vi "Scan area calc.vi"(0 "Y Width":dbl, 1 "Major Axis Direction":u16(ring) items=["Positive", "Negative"], 2 "X Width":dbl, 3 "Minor Axis Direction":u16(ring) items=["Positive", "Negative"], 4 "Scan Type":u16(ring) items=["Line Scan (Positive X)", "Line Scan (Negative X)", "Line Scan (Positive Y)", "Line Scan (Negative Y)"], 5 "Y Center":dbl, 6 "X Center":dbl) -> (7 "Y start":dbl, 8 "Y end":dbl, 9 "X end":dbl, 10 "X start":dbl)   [LabVIEW 2023]
uses:
  User_Vi/Settings.vi
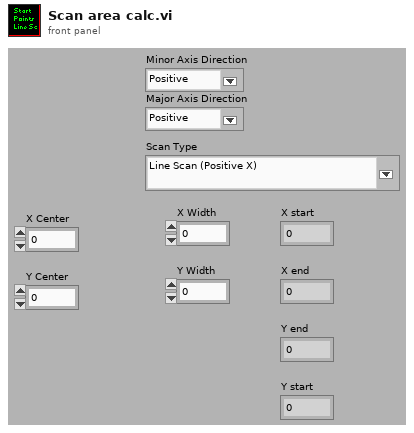
[diagram p1: front panel]
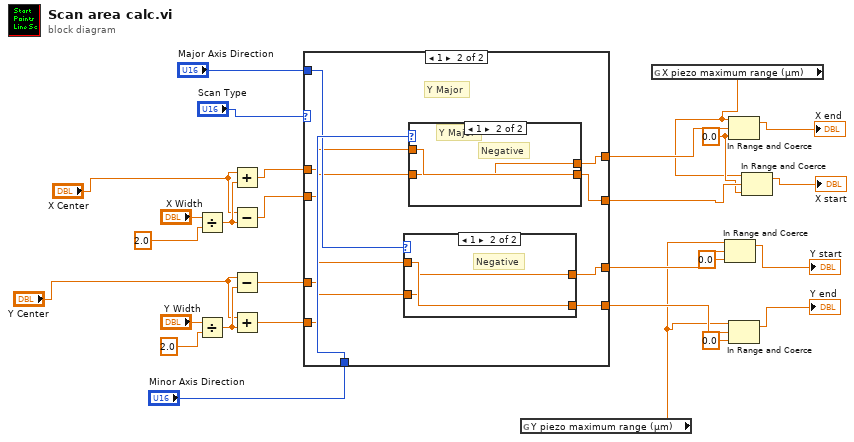
[diagram p0: block diagram]
diagram:
  w10 = 0.0 ("lower limit")
  n1 = Divide(x="X Width", y=2.0) -> (x/y=w27:dbl)
  n2 = Divide(x="Y Width", y=2.0) -> (x/y=w28:dbl)
  n3 = Add(x="X Center", y=w27) -> (x+y=w21:dbl)
  n4 = Subtract(x="X Center", y=w27) -> (x-y=w20:dbl)
  n5 = Subtract(x="Y Center", y=w28) -> (x-y=w19:dbl)
  n6 = Add(x="Y Center", y=w28) -> (x+y=w18:dbl)
  n7 = case shown="1" "Scan Type" {
    tunnel: w21 -> [w38 w52]
    tunnel: w20 -> [w37 w51]
    tunnel: [w36 w50] -> w13
    tunnel: [w35 w49] -> w11
    tunnel: w19 -> [w34 w54]
    tunnel: w18 -> [w33 w53]
    tunnel: [w32 w48] -> w7
    tunnel: [w31 w47] -> w6
    tunnel: "Major Axis Direction" -> [w30 w55]
    tunnel: "Minor Axis Direction" -> [w29 w56]
    frame 0, Default {
      # "X Major"
      n8 = case shown="1" w29 {
        tunnel: w34 -> [w40 w42]
        tunnel: w33 -> [w39 w41]
        tunnel: [w40 w41] -> w32
        tunnel: [w39 w42] -> w31
        frame 0, Default {
          # "Positive"
        }
        frame 1 {
          # "Negative"
        }
      }
      n9 = case shown="1" w30 {
        tunnel: w38 -> [w44 w45]
        tunnel: w37 -> [w43 w46]
        tunnel: [w44 w46] -> w36
        tunnel: [w43 w45] -> w35
        frame 0, Default {
          # "Positive"
        }
        frame 1 {
          # "Negative"
        }
      }
    }
    frame 1 {
      # "Y Major"
      # "Y Major"
      n10 = case shown="1" w55 {
        tunnel: w54 -> [w58 w60]
        tunnel: w53 -> [w57 w59]
        tunnel: [w58 w59] -> w48
        tunnel: [w57 w60] -> w47
        frame 0, Default {
          # "Positive"
        }
        frame 1 {
          # "Negative"
        }
      }
      n11 = case shown="1" w56 {
        tunnel: w52 -> [w62 w64]
        tunnel: w51 -> [w61 w63]
        tunnel: [w62 w63] -> w50
        tunnel: [w61 w64] -> w49
        frame 0, Default {
          # "Positive"
        }
        frame 1 {
          # "Negative"
        }
      }
    }
  }
  n12 = global read "Settings.vi" "Y piezo maximum range (µm)"() -> (w3:dbl)
  n13 = global read "Settings.vi" "X piezo maximum range (µm)"() -> (w9:dbl)
  n14 = In Range and Coerce(upper limit=w3, x=w7, lower limit=0.0) -> (coerced(x)=→"Y start":dbl)  [unwired: 1 out]
  n15 = In Range and Coerce(upper limit=w9, x=w13, lower limit=w10) -> (coerced(x)=→"X end":dbl)  [unwired: 1 out]
  n16 = In Range and Coerce(upper limit=w3, x=w6, lower limit=0.0) -> (coerced(x)=→"Y end":dbl)  [unwired: 1 out]
  n17 = In Range and Coerce(upper limit=w9, x=w11, lower limit=w10) -> (coerced(x)=→"X start":dbl)  [unwired: 1 out]
